vi "DHE_GetSyncDir2.vi"() -> (2 "sync file":path)   [LabVIEW 2016]
uses:
  DBSHAND/private/vis/DatabaseHand_Element_Get(string).vi
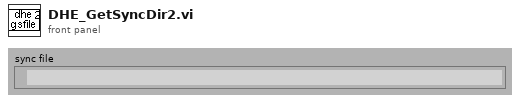
[diagram p1: front panel]
types:
  T1 = typedef "DatabaseHand_RefNum.ctl" = refnum<vi>
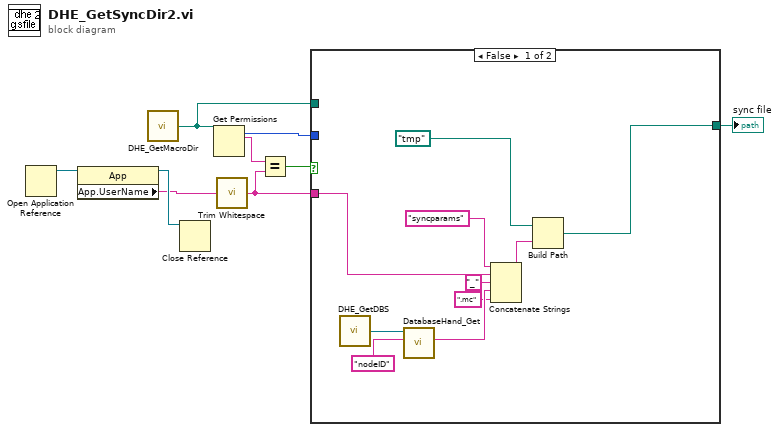
[diagram p0: block diagram]
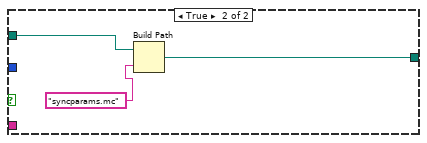
[diagram p2: hidden frame]
diagram:
  n1 = Open Application Reference() -> (3:w3:refnum<vi>)  [unwired: 1 in, 4 out]
  n2 = property class="App"(reference=w3) -> (reference out=w2:refnum<vi>, "App.UserName"=w1:string)  [unwired: 1 in, 1 out]
  n3 = call "DHE_GetMacroDir.vi"() -> ("DHE_MacroDir"=w6:path)  [unwired: 9 out]
  n4 = Close Reference(reference=w2) -> ()  [unwired: 1 in, 1 out]
  n5 = Get Permissions(11:w6) -> (2:w8:string, 5:w9:i16)  [unwired: 1 in, 3 out]
  n6 = call <vilib>:"Trim Whitespace.vi"("string"=w1) -> ("trimmed string"=w4:string)  [unwired: 1 in]
  n7 = Equal?(x=w8, y=w4) -> (x = y?=w7:bool)
  n8 = case shown="False" w7 {
    tunnel: w9 -> [_ _]
    tunnel: w6 -> [_ w22]
    tunnel: [w18 w21] -> w5
    tunnel: w4 -> [w17 _]
    frame False {
      n9 = call "DHE_GetDBS.vi"() -> ("DHE_DBSRef"=w15:T1)  [unwired: 9 out]
      n10 = call-poly "DatabaseHand_Get.vi"("name"="nodeID", "Database RefNum in"=w15) -> ("value"=w12:string)  [unwired: 3 in, 6 out]
      n11 = Concatenate Strings("syncparams" ("name or relative path"), w17, "_" ("string"), w12, ".mc" ("string")) -> (w19:string)
      n12 = Build Path(base path=path "/tmp", name or relative path=w19) -> (appended path=w18:path)
    }
    frame True {
      n13 = Build Path(base path=w22, name or relative path="syncparams.mc") -> (appended path=w21:path)
    }
  }
  "sync file" <- w5
